vi "Calibrate Stereo Vision System.vi"() -> ()   [LabVIEW 2019]
doc: "This example acquires images and demonstrates the binocular stereo vision algorithms installed with NI Vision Development Module. This example requires NI-IMAQdx. Refer to the Detailed Help for more information."
uses:
  SubVIs/Stereo - Calibration Manager Function.ctl
  <vilib>/vision/Stereo.llb/IMAQ Binocular Reference Coordinate System.ctl
  SubVIs/Stereo - Global Variables.vi
  <vilib>/vision/NI_Vision_Development_Module.lvlib
panel:
  in  "Process Band":bool
  out "Unit":string
  in  "Units":string[](array[string])=["", "Angström", "Micrometer", "Millimeter", "Centimeter", "Meter", "Kilometer", "Microinch", "Inch", "Feet", "Nautical miles", "Standard miles", "Steps"]
  out "Depth":dbl caption="Depth:"
  in  "Interpolate Disparity":bool=TRUE
  in  "Overlay Horizontal Lines":bool
  in  "View":enum16{"Acquired Images", "Rectified Images"}(ring)
  out "Grid Descriptor":cluster{"X Step":sgl, "Y Step":sgl, "Unit":T1}={"X Step"=1.0, "Y Step"=1.0, "Unit"=enum."Inch"}
  out "Grid Size":cluster{"X":i32, "Y":i32}
  in  "Live Image":bool=TRUE
  out "Calibration Status":u16(ring)
  in  "Display":enum16{"Disparity Image", "Depth Image"}(ring)
  in  "Relative Coordinate System":T2
  out "Image":sgl[][](graph) caption="Grid Coverage"
  in  "Exit":bool
  in  "Tab Control":T3(tab)
  out "Grid Coverage":T5
  in  "Save Single Calibrations":bool
  out "Quality":T6 caption="Stereo Calibration Quality" {"Rectification Quality 2" format="%#.5g"; "Rectification Quality" format="%#.5g"; "Calibration Quality" format="%#.5g"; "Max Distance" format="%#.4g"}
  in  "Save Grid Images":bool
  out "Scrollbar":u8(slide) caption="Acquire image in..." max=50 scale=0.0..100.0
  in  "Save Stereo Calibration":bool
  in  "Scaling Factor":sgl=1.0 min=0 max=1 step=0.1
  in  "Load":bool
  in  "Calibrate":bool
  out "Instruction Images":u16(ring) caption="Grid Orientation"
  out "Instructions":string
  in  "Time Lapse":u16=4 caption="Image Acquisition Time Lapse" min=1 max=60 step=1
  out "Grid Valid":bool=TRUE
  out "Calibration Grids":cluster{"Left Image":T4, "Right Image":T4}[](array[cluster]) caption="Left Calibration Grids"
  in  "Show":enum16{"Grid Coverage", "Calibration Grids"}(ring)
  in  "Max Depth (SGBM)":sgl=45.0 caption="Maximum Depth"
  in  "Correspondence Options SGBM":T7={"Method"=0, "Window Size"=15.0, "Minimum Disparity"=0.0, "Number of Disparity"=144.0, "P1"=100.0, "P2"=500.0, "Full DP"=FALSE, "Max Left Right Disparity"=5.0, "Subpixel"=TRUE, "Invalid Disparity Replace Value"=-16.0} caption="Correspondence Options" {"Method" items=["SAD"]; "Number of Disparity" min=16.0 step=16.0; "Window Size" min=5.0 max=255.0 step=2.0}
  in  "Postfilter Options SGBM":T8={"Texture Threshold"=0.0, "Uniqueness Ratio"=0.0, "Speckle Window Size"=5.0, "Speckle Range"=200.0} caption="Postfilter Options" {"Speckle Range" min=0.0; "Speckle Window Size" min=0.0; "Uniqueness Ratio" min=0.0 max=100.0; "Texture Threshold" min=0.0}
  in  "Filter Cap":u32=32
  in  "Correspondence Options BM":T9={"Method"=0, "Window Size"=25.0, "Minimum Disparity"=0.0, "Number of Disparity"=144.0, "Left - Right Check"=5.0, "Subpixel"=TRUE, "Invalid Disparity Replace Value"=-16.0} caption="Correspondence Options" {"Method" items=["SAD"]; "Number of Disparity" min=16.0 step=16.0; "Window Size" min=5.0 max=255.0 step=2.0}
  in  "Postfilter Options BM":T8={"Texture Threshold"=0.0, "Uniqueness Ratio"=0.0, "Speckle Window Size"=5.0, "Speckle Range"=200.0} caption="Postfilter Options" {"Speckle Range" min=0.0; "Speckle Window Size" min=0.0; "Uniqueness Ratio" min=0.0 max=100.0 step=1.0; "Texture Threshold" min=0.0}
  in  "Prefilter Options":T10={"Filter Type"=2, "Filter Size"=9.0, "Filter Cap"=31.0} {"Filter Type" items=["None", "Normal Response", "Sobel"]; "Filter Cap" min=1.0 max=63.0 step=1.0; "Filter Size" min=5.0 max=255.0 step=2.0}
  in  "Max Depth (BM)":sgl=45.0 caption="Maximum Depth"
  out "Right Image":T4(plugin-control)
  out "Left Image":T4(plugin-control)
  # "Overview: Demonstrate how to calibrate a stereo system and compute a depth image.\nRequirements: LabVIEW Full Development System, NI-IMAQdx and Vision Development Module\nNote: This example does not run on LabVIEW Real Time"
  # "s"
  # "Right Calibration Grids"
  # "Set the Maximum Depth corresponding to your setting:"
  # "Set the Maximum Depth corresponding to your setting:"
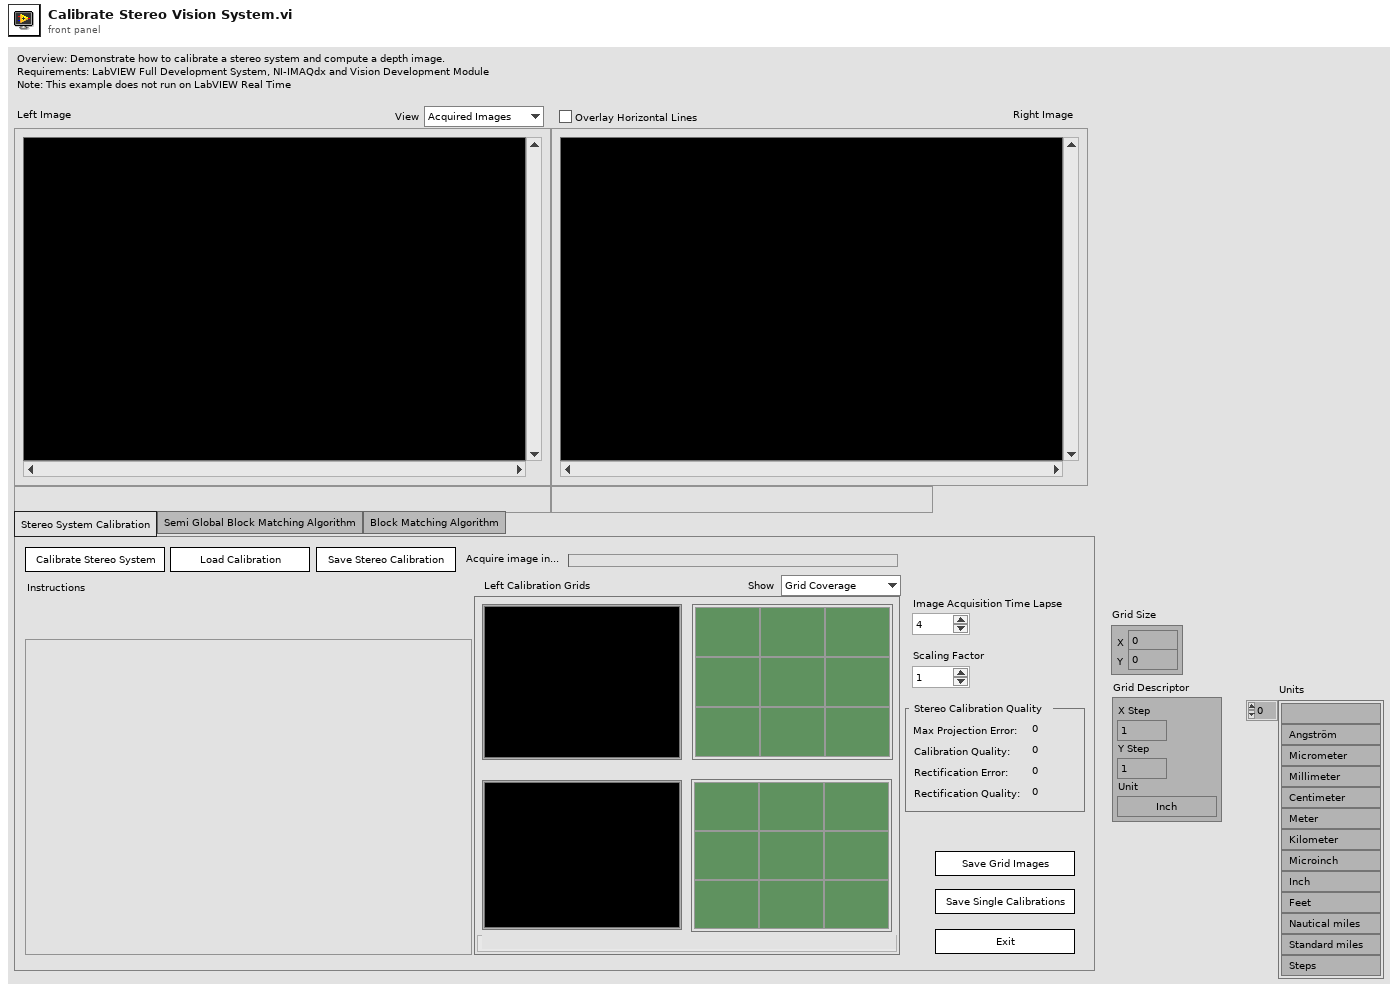
[diagram p1: front panel]
types:
  T1 = typedef "Image Unit" = enum32{"Undefined", "Angström", "Micrometer", "Millimeter", "Centimeter", "Meter", "Kilometer", "Microinch", "Inch", "Feet", "Nautical miles", "Standard miles", "Steps"}
  T2 = cluster{"Translation":cluster{"X":dbl, "Y":dbl, "Z":dbl}, "Rotation":cluster{"X":dbl, "Y":dbl, "Z":dbl}}
  T3 = enum32{"Stereo System Calibration", "Semi Global Block Matching Algorithm", "Block Matching Algorithm"}
  T4 = typedef "IMAQ Image.ctl" = refnum<image>
  T5 = cluster{"Left Image":T4, "Left Grid Coverage":bool[][], "Left Grid Coverage 3":string[][], "Right Image":T4, "Left Grid Coverage 2":bool[][], "Left Grid Coverage 4":string[][]}
  T6 = cluster{"Max Distance":dbl, "Calibration Quality":dbl, "Rectification Quality":dbl, "Rectification Quality 2":dbl}
  T7 = cluster{"Method":u16, "Window Size":dbl, "Minimum Disparity":dbl, "Number of Disparity":dbl, "P1":dbl, "P2":dbl, "Full DP":bool, "Max Left Right Disparity":dbl, "Subpixel":bool, "Invalid Disparity Replace Value":dbl}
  T8 = cluster{"Texture Threshold":dbl, "Uniqueness Ratio":dbl, "Speckle Window Size":dbl, "Speckle Range":dbl}
  T9 = cluster{"Method":u16, "Window Size":dbl, "Minimum Disparity":dbl, "Number of Disparity":dbl, "Left - Right Check":dbl, "Subpixel":bool, "Invalid Disparity Replace Value":dbl}
  T10 = cluster{"Filter Type":u16, "Filter Size":dbl, "Filter Cap":dbl}
  T11 = typedef "Stereo - Calibration Manager Function.ctl" = enum16{"Init", "Add Grid Images", "Get Images", "Dispose"}
  T12 = enum32{"Zero Order", "Bilinear", "Quadratic", "Cubic", "Bilinear Fixed"}
  T13 = typedef "IMAQ Binocular Reference Coordinate System.ctl" = enum32{" Left Camera", "Right Camera"}
  T14 = cluster{"Learn Lookup Table?":bool, "Render to original image?":bool, "Scaling Factor":sgl}
  T15 = enum8{"Enabled", "Disabled", "Disabled and Grayed Out"}
  T16 = enum32{"Page Enabled", "Page Disabled", "Page Disabled & Grayed"}
  T17 = typedef "Image Type" = u32
  T18 = typedef "IMAQ Binocular Stereo Session.ctl" = refnum<k1>
  T19 = typedef "Calibration Reference Points.ctl" = cluster{"Pixel Coordinates":cluster{"X":dbl, "Y":dbl}[], "Real World Coordinates":cluster{"X":dbl, "Y":dbl}[], "Unit":T1, "Image Size":cluster{"X":u32, "Y":u32}}
  T20 = cluster{"Image (dup)":T4, "Reference Points":T19}
  T21 = cluster{"Max. Projection Error":dbl, "Calibration Quality":dbl, "Max. Rectification Error":dbl, "Rectification Quality":dbl}
  T22 = typedef "LVPoint32TypeDef.ctl" = cluster{"Horizontal":i32, "Vertical":i32}
  T23 = cluster{"Max Depth (BM)":sgl, "Max Depth (BM)":sgl}
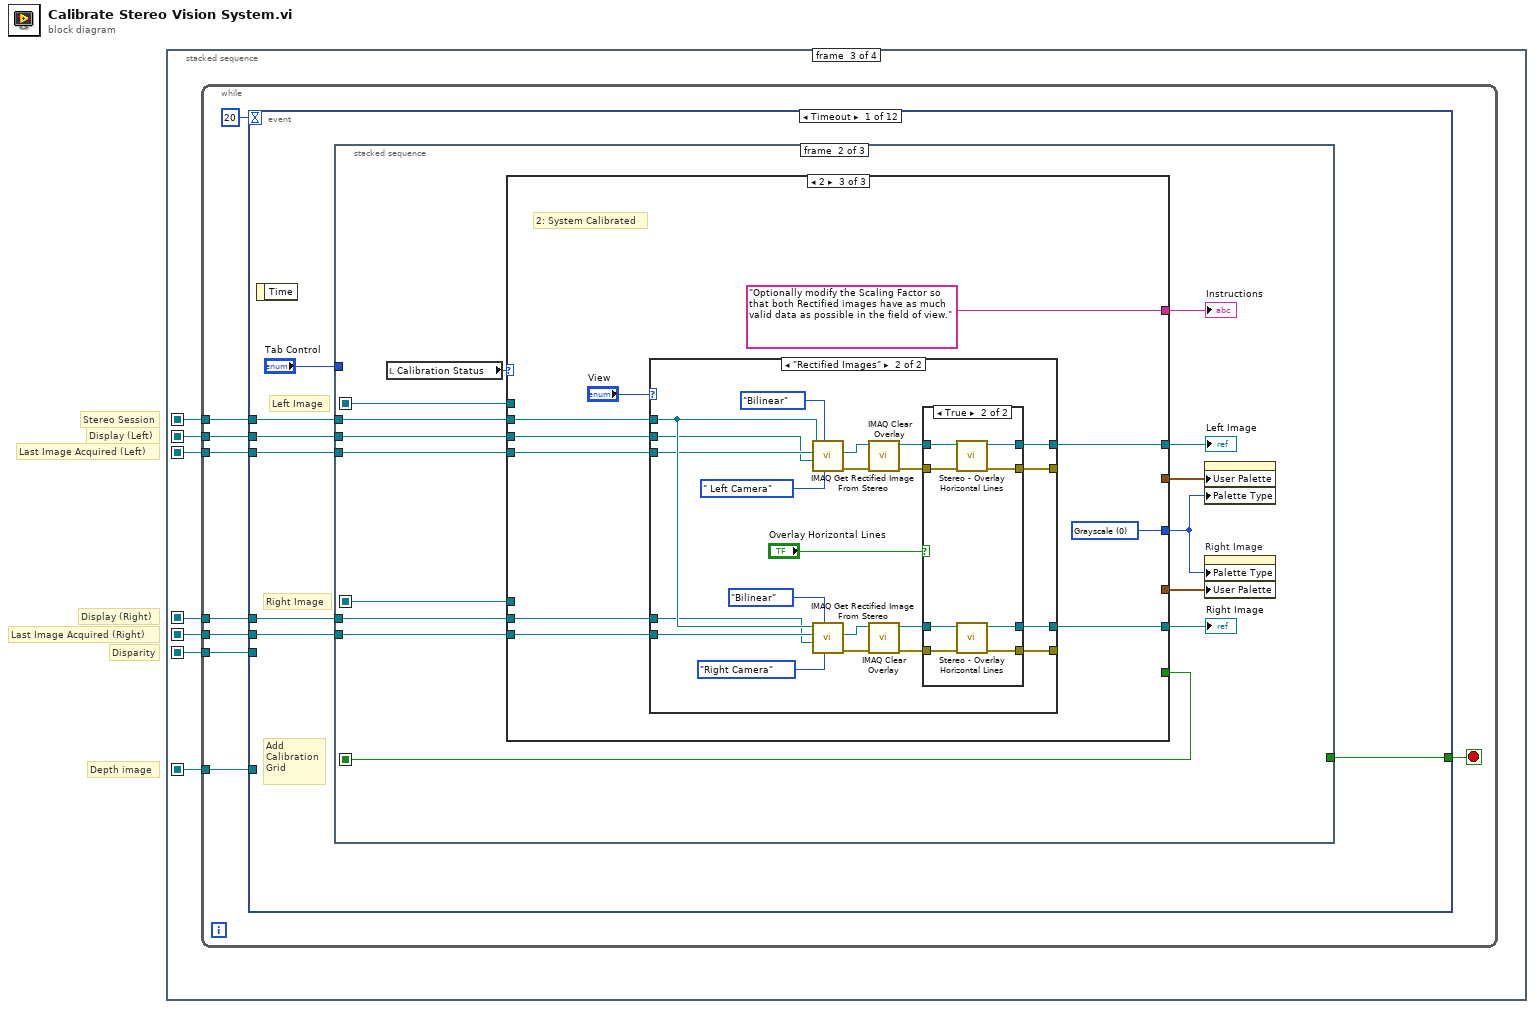
[diagram p0: block diagram]
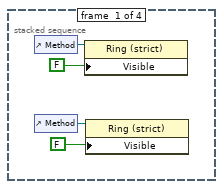
[diagram p2: hidden frame]
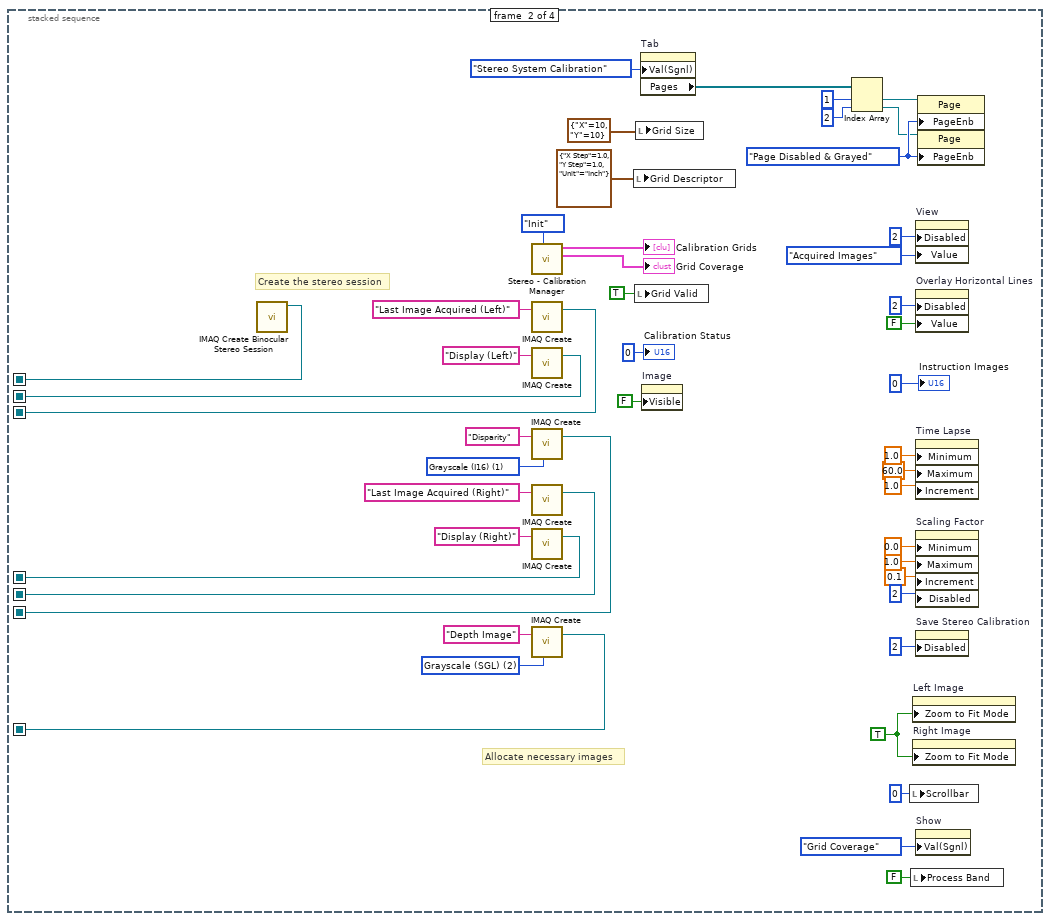
[diagram p3: hidden frame]
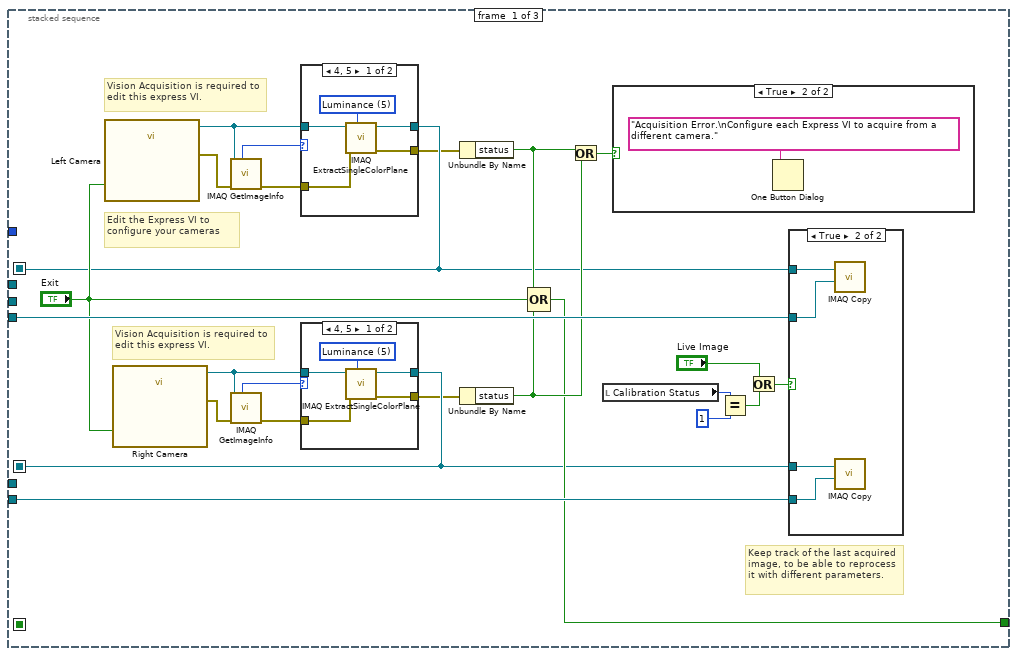
[diagram p4: hidden frame]
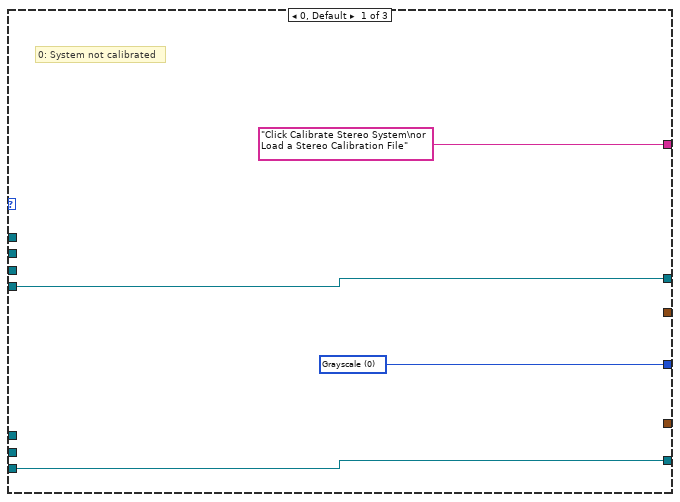
[diagram p9: hidden frame]
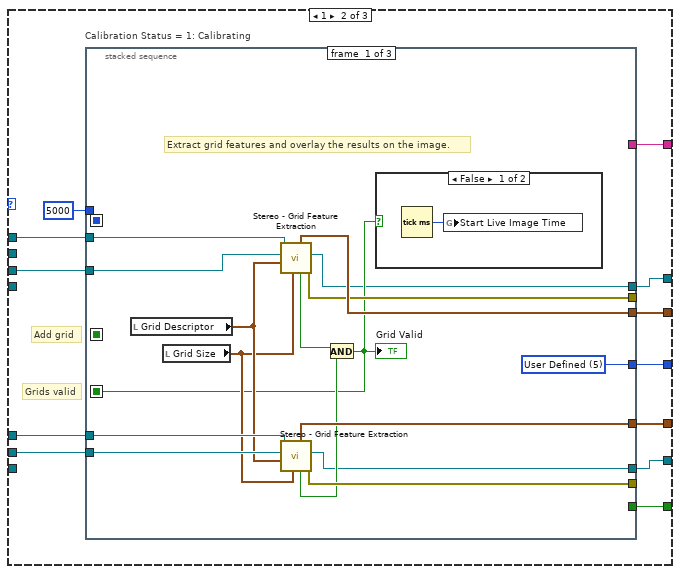
[diagram p10: hidden frame]
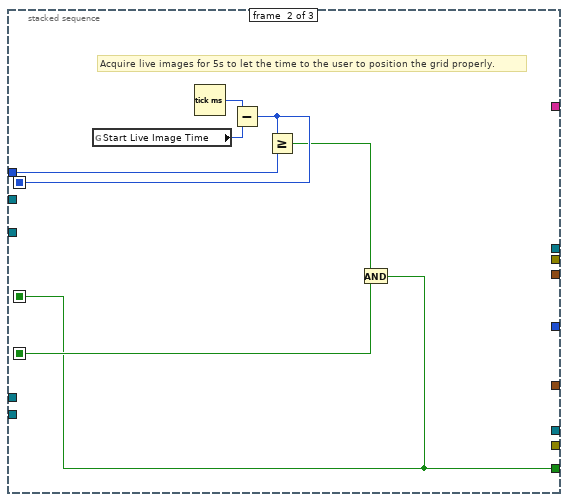
[diagram p12: hidden frame]
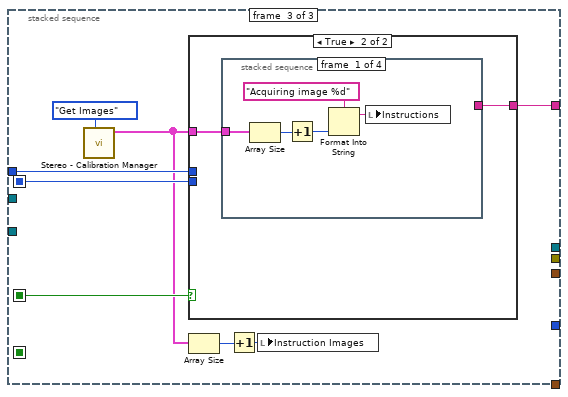
[diagram p13: hidden frame]
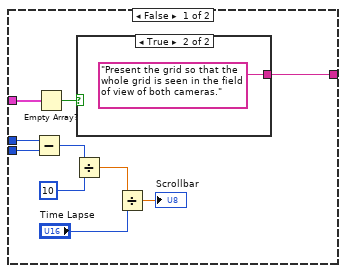
[diagram p14: hidden frame]
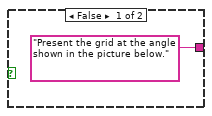
[diagram p15: hidden frame]
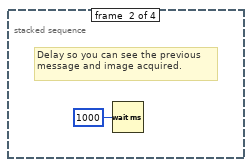
[diagram p16: hidden frame]
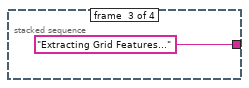
[diagram p17: hidden frame]
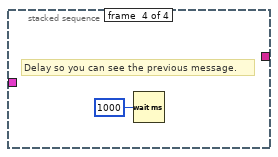
[diagram p18: hidden frame]
diagram:
  # "Depth image"
  # "Last Image Acquired (Right)"
  # "Disparity"
  # "Display (Right)"
  # "Display (Left)"
  # "Last Image Acquired (Left)"
  # "Stereo Session"
  n1 = stacked-sequence {
    seq-local: [_ w49 _ _] -> [_ _ w58 w606]
    seq-local: [_ w48 _ _] -> [_ _ w57 w604]
    seq-local: [_ w47 _ _] -> [_ _ w56 w607]
    seq-local: [_ w42 _ _] -> [_ _ w54 w603]
    seq-local: [_ w43 _ _] -> [_ _ w55 w605]
    seq-local: [_ w40 _ _] -> [_ _ w53 w602]
    seq-local: [_ w36 _ _] -> [_ _ w52 w600]
    frame #0 {
      n2 = control-ref of="Method"() -> (w4:refnum<vi>)
      n3 = control-ref of="Method"() -> (w1:refnum<vi>)
      n4 = property class="Ring (strict)"(reference=w4, "Visible"=FALSE) -> ()  [unwired: 1 in, 2 out]
      n5 = property class="Ring (strict)"(reference=w1, "Visible"=FALSE) -> ()  [unwired: 1 in, 2 out]
    }
    frame #1 {
      w12 = TRUE ("Zoom to Fit Mode")
      w30 = T16."Page Disabled & Grayed" ("Page Enabled State")
      w37 = T17 2 items=["Grayscale (U8)", "Grayscale (I16)", "Grayscale (SGL)", "Complex (CSG)", "RGB (U32)", "HSL (U32)", "RGB (U64)", "Grayscale (U16)"] ("Image Type")
      w39 = T17 1 items=["Grayscale (U8)", "Grayscale (I16)", "Grayscale (SGL)", "Complex (CSG)", "RGB (U32)", "HSL (U32)", "RGB (U64)", "Grayscale (U16)"] ("Image Type")
      # "Allocate necessary images"
      # "Create the stereo session"
      n6 = call "IMAQ Create Binocular Stereo Session"() -> ("Binocular Stereo Session Out"=w47:T18)  [unwired: 1 in, 10 out]
      n7 = call "Stereo - Calibration Manager.vi"("Function"=Stereo_-_Calibration_Manager_Function."Init") -> ("Grid Coverage"=→"Grid Coverage":T5, "Grid Images out"=→"Calibration Grids":cluster{"Left Image":T4, "Right Image":T4}[])  [unwired: 2 in, 7 out]
      n8 = call "IMAQ Create"("Image Name"="Last Image Acquired (Left)") -> ("New Image"=w43:T4)  [unwired: 3 in, 2 out]
      n9 = call "IMAQ Create"("Image Name"="Display (Left)") -> ("New Image"=w49:T4)  [unwired: 3 in, 2 out]
      n10 = call "IMAQ Create"("Image Name"="Disparity", "Image Type"=w39) -> ("New Image"=w40:T4)  [unwired: 2 in, 2 out]
      n11 = call "IMAQ Create"("Image Name"="Last Image Acquired (Right)") -> ("New Image"=w42:T4)  [unwired: 3 in, 2 out]
      n12 = call "IMAQ Create"("Image Name"="Display (Right)") -> ("New Image"=w48:T4)  [unwired: 3 in, 2 out]
      n13 = call "IMAQ Create"("Image Name"="Depth Image", "Image Type"=w37) -> ("New Image"=w36:T4)  [unwired: 2 in, 2 out]
      n14 = local write "Grid Descriptor"(cluster{"X Step":sgl, "Y Step":sgl, "Unit":T1} {"X Step"=1.0, "Y Step"=1.0, "Unit"=enum."Inch"} ("Grid Descriptor")) -> ()
      n15 = local write "Grid Valid"(TRUE ("Grid Valid")) -> ()
      n16 = local write "Grid Size"(cluster{"X":i32, "Y":i32} {"X"=10, "Y"=10} ("Grid Size")) -> ()
      n17 = property on="Tab" class="TabCtl (strict)"("Val(Sgnl)"=T3."Stereo System Calibration" ("Value (Signaling)")) -> ("Pages"=w34:refnum<vi>[])  [unwired: 2 in, 2 out]
      n18 = property on="Image" class="IntGraph (strict)"("Visible"=FALSE) -> ()  [unwired: 2 in, 2 out]
      n19 = Index Array(array=w34, index #1=1 ("index"), index #2=2 ("index")) -> (element #1=w33:refnum<vi>, element #2=w29:refnum<vi>)
      n20 = local write "Scrollbar"(u8 0 ("Scrollbar")) -> ()
      n21 = local write "Process Band"(FALSE ("Process Band")) -> ()
      n22 = property on="Left Image" class="ImageControl"("Zoom to Fit Mode"=w12) -> ()  [unwired: 2 in, 2 out]
      n23 = property on="Right Image" class="ImageControl"("Zoom to Fit Mode"=w12) -> ()  [unwired: 2 in, 2 out]
      n24 = property on="View" class="Enum (strict)"("Disabled"=u8 2, "Value"=enum16{"Acquired Images", "Rectified Images"}."Acquired Images" ("View")) -> ()  [unwired: 2 in, 2 out]
      n25 = property on="Overlay Horizontal Lines" class="Bool (strict)"("Disabled"=u8 2, "Value"=FALSE ("Overlay Horizontal Lines")) -> ()  [unwired: 2 in, 2 out]
      n26 = property on="Time Lapse" class="DigNum (strict)"("Minimum"=1.0 ("Data Entry Limits:Minimum"), "Maximum"=60.0 ("Data Entry Limits:Maximum"), "Increment"=1.0 ("Data Entry Limits:Increment")) -> ()  [unwired: 2 in, 2 out]
      n27 = property on="Scaling Factor" class="DigNum (strict)"("Minimum"=0.0 ("Data Entry Limits:Minimum"), "Maximum"=1.0 ("Data Entry Limits:Maximum"), "Increment"=0.1 ("Data Entry Limits:Increment"), "Disabled"=u8 2) -> ()  [unwired: 2 in, 2 out]
      n28 = property on="Save Stereo Calibration" class="Bool"("Disabled"=u8 2) -> ()  [unwired: 2 in, 2 out]
      n29 = property on="Show" class="Enum (strict)"("Val(Sgnl)"=enum16{"Grid Coverage", "Calibration Grids"}."Grid Coverage" ("Value (Signaling)")) -> ()  [unwired: 2 in, 2 out]
      n30 = property class="Page"(reference=w33, "PageEnb"=w30) -> ()  [unwired: 1 in, 2 out]
      n31 = property class="Page"(reference=w29, "PageEnb"=w30) -> ()  [unwired: 1 in, 2 out]
      "Calibration Status" <- u16 0 ("Status")
      "Instruction Images" <- u16 0 ("Grid Orientation")
    }
    frame #2 {
      n32 = while {
        tunnel: w58 -> [w66]
        tunnel: w57 -> [w65]
        tunnel: w56 -> [w63]
        tunnel: w55 -> [w62]
        tunnel: w54 -> [w61]
        tunnel: w53 -> [w60]
        tunnel: w52 -> [w59]
        stop <- w67 stop-if-true
        n33 = event shown="[0] Timeout" {
          selector: _ -> [_ _ _ _ _ _ _ _ _ _ _ _]
          dyn-events: _ -> [_ _ _ _ _ _ _ _ _ _ _ _]
          timeout: 20 -> [_ _ _ _ _ _ _ _ _ _ _ _]
          tunnel: [w74 _ _ _ _ _ _ _ _ _ _ _] -> w67
          tunnel: w66 -> [w73 _ _ _ _ _ _ _ _ _ _ _]
          tunnel: w65 -> [w72 _ _ _ _ _ _ _ _ _ _ _]
          tunnel: w63 -> [w69 _ _ w328 w377 w391 _ _ _ w455 _ w591]
          tunnel: w62 -> [w71 _ _ _ _ _ _ _ _ w454 _ _]
          tunnel: w61 -> [w70 _ _ _ _ _ _ _ _ w453 _ _]
          tunnel: w60 -> [_ _ _ _ _ _ _ _ _ w452 _ w590]
          tunnel: w59 -> [_ _ _ _ _ _ _ _ _ w445 _ _]
          event Timeout {
            # "Add\nCalibration\nGrid"
            # "Right Image"
            # "Left Image"
            n34 = event-data() -> ()  [unwired: 2 out]
            n35 = stacked-sequence {
              seq-local: [w82 _ _] -> [_ w129 w254]
              seq-local: [w77 _ _] -> [_ w127 w253]
              seq-local: [_ w131 _] -> [_ _ w250]
              tunnel: [w87 _ _] -> w74
              tunnel: w73 -> [_ w128 w252]
              tunnel: w72 -> [_ w126 w251]
              tunnel: w71 -> [w98 w120 _]
              tunnel: w70 -> [w97 w119 _]
              tunnel: w69 -> [_ w118 _]
              tunnel: "Tab Control" -> [_ _ w249]
              frame #0 {
                # "Vision Acquisition is required to edit this express VI."
                # "Vision Acquisition is required to edit this express VI."
                # "Edit the Express VI to configure your cameras"
                # "Keep track of the last acquired image, to be able to reprocess it with different parameters."
                n36 = call "Left Camera"("Stop (F)"="Exit") -> ("Image Out"=w83:T4, "error out"=w86:errorcluster)  [unwired: 1 in, 24 out]
                n37 = call "Right Camera"("Stop (F)"="Exit") -> ("Image Out"=w78:T4, "error out"=w85:errorcluster)  [unwired: 1 in, 24 out]
                n38 = call "IMAQ GetImageInfo"("error in (no error)"=w86, "Image"=w83) -> ("error out"=w81:errorcluster, "Image Type"=w84:T17)  [unwired: 8 out]
                n39 = call "IMAQ GetImageInfo"("error in (no error)"=w85, "Image"=w78) -> ("error out"=w79:errorcluster, "Image Type"=w75:T17)  [unwired: 8 out]
                n40 = case shown="4, 5" w84 {
                  tunnel: w83 -> [w110 w112]
                  tunnel: [w108 w112] -> w82
                  tunnel: w81 -> [w107 w111]
                  tunnel: [w106 w111] -> w80
                  frame 4, 5 {
                    w109 = 5 items=["Red", "Green", "Blue", "Hue", "Saturation", "Luminance", "Value", "Intensity"] ("Color Plane")
                    n41 = call "IMAQ ExtractSingleColorPlane"("Color Plane"=w109, "error in (no error)"=w107, "Image Src"=w110) -> ("error out"=w106:errorcluster, "Image Dst Out"=w108:T4)  [unwired: 1 in, 6 out]
                  }
                  frame Default {
                  }
                }
                n42 = case shown="4, 5" w75 {
                  tunnel: w78 -> [w103 w105]
                  tunnel: [w101 w105] -> w77
                  tunnel: w79 -> [w100 w104]
                  tunnel: [w99 w104] -> w76
                  frame 4, 5 {
                    w102 = 5 items=["Red", "Green", "Blue", "Hue", "Saturation", "Luminance", "Value", "Intensity"] ("Color Plane")
                    n43 = call "IMAQ ExtractSingleColorPlane"("Color Plane"=w102, "error in (no error)"=w100, "Image Src"=w103) -> ("error out"=w99:errorcluster, "Image Dst Out"=w101:T4)  [unwired: 1 in, 6 out]
                  }
                  frame Default {
                  }
                }
                n44 = Unbundle By Name(w80) -> ("status"=w89:bool)
                n45 = Unbundle By Name(w76) -> ("status"=w88:bool)
                n46 = Compound Arithmetic op=OR(w89, "Exit", w88) -> (w87:bool)
                n47 = Or(x=w89, y=w88) -> (x .or. y?=w91:bool)
                n48 = local read "Calibration Status"() -> (w96:u16)
                n49 = case shown="True" w91 {
                  frame False {
                  }
                  frame True {
                    n50 = One Button Dialog(message="Acquisition Error.\nConfigure each Express VI to acquire from a different camera.") -> ()  [unwired: 2 out]
                  }
                }
                n51 = Equal?(x=w96, y=u16 1) -> (x = y?=w93:bool)
                n52 = Or(x="Live Image", y=w93) -> (x .or. y?=w92:bool)
                n53 = case shown="True" w92 {
                  tunnel: w82 -> [_ w117]
                  tunnel: w98 -> [_ w116]
                  tunnel: w77 -> [_ w115]
                  tunnel: w97 -> [_ w114]
                  frame False {
                  }
                  frame True {
                    n54 = call "IMAQ Copy"("Image Dst"=w116, "Image Src"=w117) -> ()  [unwired: 1 in, 5 out]
                    n55 = call "IMAQ Copy"("Image Dst"=w114, "Image Src"=w115) -> ()  [unwired: 1 in, 5 out]
                  }
                }
              }
              frame #1 {
                n56 = local read "Calibration Status"() -> (w130:u16)
                n57 = case shown="2" w130 {
                  tunnel: ["Click Calibrate Stereo System\nor Load a Stereo Calibration File" ("Instructions") w148 "Optionally modify the Scaling Factor so that both Rectified images have as much valid data as possible in the field of view." ("Instructions")] -> w132
                  tunnel: [_ w147 _] -> w131
                  tunnel: w129 -> [_ w146 _]
                  tunnel: w128 -> [_ w145 w205]
                  tunnel: w127 -> [_ w144 _]
                  tunnel: w126 -> [_ w143 w204]
                  tunnel: [w135 w142 w209] -> w122
                  tunnel: [w134 w141 w207] -> w123
                  tunnel: [_ w140 _] -> w125
                  tunnel: [_ w139 _] -> w124
                  tunnel: [w136 w138 w212] -> w121
                  tunnel: w120 -> [w135 _ w210]
                  tunnel: w119 -> [w134 _ w208]
                  tunnel: w118 -> [_ _ w206]
                  frame 0, Default {
                    w136 = u32 0 items=["Grayscale", "Binary", "Gradient", "Rainbow", "Temperature", "User Defined"] ("Palette:Palette Type")
                    # "0: System not calibrated"
                  }
                  frame 1 {
                    # "Add grid"
                    # "Grids valid"
                    n58 = stacked-sequence "Calibration Status = 1: Calibrating" {
                      seq-local: [w151 _ _] -> [_ w167 _]
                      seq-local: [_ w166 _] -> [_ _ w180]
                      seq-local: [_ w169 _] -> [_ _ w178]
                      tunnel: [_ _ w177] -> w148
                      tunnel: [_ w166 _] -> w147
                      tunnel: w146 -> [w164 _ _]
                      tunnel: w145 -> [w163 _ _]
                      tunnel: w144 -> [w162 _ _]
                      tunnel: w143 -> [w161 _ _]
                      tunnel: [w150 _ _] -> w142
                      tunnel: [w149 _ _] -> w141
                      tunnel: [w160 _ _] -> w140
                      tunnel: [w159 _ _] -> w139
                      tunnel: [w158 _ _] -> w138
                      tunnel: [w157 _ _] -> _
                      tunnel: [w156 _ _] -> _
                      tunnel: u32 5000 ("y") -> [_ w170 w179]
                      frame #0 {
                        w158 = u32 5 items=["Grayscale", "Binary", "Gradient", "Rainbow", "Temperature", "User Defined"] ("Palette:Palette Type")
                        # "Extract grid features and overlay the results on the image."
                        n59 = local read "Grid Descriptor"() -> (w155:cluster{"X Step":sgl, "Y Step":sgl, "Unit":T1})
                        n60 = local read "Grid Size"() -> (w154:cluster{"X":i32, "Y":i32})
                        n61 = call "Stereo - Grid Feature Extraction.vi"("Grid Size"=w154, "Grid Descriptor"=w155, "Display Image in"=w163, "Image in"=w164) -> ("error out"=w157:errorcluster, "Display Image out"=w150:T4, "Valid Grid"=w153:bool, "Color Palette"=w159:cluster{"Red":u8, "Green":u8, "Blue":u8}[])  [unwired: 2 in, 2 out]
                        n62 = call "Stereo - Grid Feature Extraction.vi"("Grid Size"=w154, "Grid Descriptor"=w155, "Display Image in"=w161, "Image in"=w162) -> ("error out"=w156:errorcluster, "Display Image out"=w149:T4, "Valid Grid"=w152:bool, "Color Palette"=w160:cluster{"Red":u8, "Green":u8, "Blue":u8}[])  [unwired: 2 in, 2 out]
                        n63 = And(x=w153, y=w152) -> (x .and. y?=w151:bool)
                        "Grid Valid" <- w151
                        n64 = case shown="False" w151 {
                          frame False {
                            n65 = Tick Count (ms)() -> (millisecond timer value=w165:u32)
                            n66 = global write "Stereo - Global Variables.vi" "Start Live Image Time"(w165) -> ()
                          }
                          frame True {
                          }
                        }
                      }
                      frame #1 {
                        # "Acquire live images for 5s to let the time to the user to position the grid properly."
                        n67 = global read "Stereo - Global Variables.vi" "Start Live Image Time"() -> (w171:u32)
                        n68 = Tick Count (ms)() -> (millisecond timer value=w172:u32)
                        n69 = Subtract(x=w172, y=w171) -> (x-y=w169:u32)
                        n70 = Greater Or Equal?(x=w169, y=w170) -> (x >= y?=w168:bool)
                        n71 = And(x=w168, y=w167) -> (x .and. y?=w166:bool)
                      }
                      frame #2 {
                        n72 = call "Stereo - Calibration Manager.vi"("Function"=Stereo_-_Calibration_Manager_Function."Get Images") -> ("Grid Images out"=w173:cluster{"Left Image":T4, "Right Image":T4}[])  [unwired: 2 in, 8 out]
                        n73 = case shown="True" w180 {
                          tunnel: w178 -> [w189 _]
                          tunnel: w179 -> [w190 _]
                          tunnel: [w181 w194] -> w177
                          tunnel: w173 -> [w186 w193]
                          frame False {
                            n74 = Subtract(x=w190, y=w189) -> (x-y=w188:u32)
                            n75 = Empty Array?(array=w186) -> (empty?=w185:bool)
                            n76 = Divide(x=w188, y=u32 10) -> (x/y=w183:dbl)
                            n77 = case shown="True" w185 {
                              tunnel: ["Present the grid at the angle shown in the picture below." ("Instructions") "Present the grid so that the whole grid is seen in the field of view of both cameras." ("Instructions")] -> w181
                              frame False {
                              }
                              frame True {
                              }
                            }
                            n78 = Divide(x=w183, y="Time Lapse") -> (x/y=→"Scrollbar":dbl)
                          }
                          frame True {
                            n79 = stacked-sequence {
                              tunnel: [_ _ "Extracting Grid Features..." ("Instructions") _] -> w194
                              tunnel: w193 -> [w195 _ _ _]
                              frame #0 {
                                n80 = Array Size(array=w195) -> (size(s)=w199:i32)
                                n81 = Increment(x=w199) -> (x+1=w197:i32)
                                n82 = Format Into String(format string="Acquiring image %d" ("Instructions"), w197) -> (resulting string=w196:string)  [unwired: 2 in, 1 out]
                                n83 = local write "Instructions"(w196) -> ()
                              }
                              frame #1 {
                                # "Delay so you can see the previous message and image acquired."
                                n84 = Wait (ms)(milliseconds to wait=u32 1000) -> ()  [unwired: 1 out]
                              }
                              frame #2 {
                              }
                              frame #3 {
                                # "Delay so you can see the previous message."
                                n85 = Wait (ms)(milliseconds to wait=u32 1000) -> ()  [unwired: 1 out]
                              }
                            }
                          }
                        }
                        n86 = Array Size(array=w173) -> (size(s)=w175:i32)
                        n87 = Increment(x=w175) -> (x+1=w174:i32)
                        n88 = local write "Instruction Images"(w174) -> ()
                      }
                    }
                  }
                  frame 2 {
                    w212 = u32 0 items=["Grayscale", "Binary", "Gradient", "Rainbow", "Temperature", "User Defined"] ("Palette:Palette Type")
                    # "2: System Calibrated"
                    n89 = case shown="\"Rectified Images\"" "View" {
                      tunnel: w210 -> [w213 w233]
                      tunnel: [w213 w228] -> w209
                      tunnel: w208 -> [w214 w232]
                      tunnel: [w214 w227] -> w207
                      tunnel: w206 -> [_ w236]
                      tunnel: w205 -> [_ w231]
                      tunnel: w204 -> [_ w230]
                      tunnel: [_ w229] -> _
                      tunnel: [_ w226] -> _
                      frame "Acquired Images", Default {
                      }
                      frame "Rectified Images" {
                        n90 = call "IMAQ Get Rectified Image From Stereo"("Reference Coordinate System"=IMAQ_Binocular_Reference_Coordinate_System." Left Camera", "Interpolation Type"=T12."Bilinear", "Image Dst"=w231, "Image Src"=w233, "Binocular Stereo Session"=w236) -> ("error out"=w224:errorcluster, "Image Dst Out"=w222:T4)  [unwired: 1 in, 4 out]
                        n91 = call "IMAQ Get Rectified Image From Stereo"("Reference Coordinate System"=IMAQ_Binocular_Reference_Coordinate_System."Right Camera", "Interpolation Type"=T12."Bilinear", "Image Dst"=w230, "Image Src"=w232, "Binocular Stereo Session"=w236) -> ("error out"=w218:errorcluster, "Image Dst Out"=w220:T4)  [unwired: 1 in, 4 out]
                        n92 = call "IMAQ Clear Overlay"("error in (no error)"=w224, "Image"=w222) -> ("error out"=w223:errorcluster, "Image Out"=w221:T4)  [unwired: 1 in, 7 out]
                        n93 = call "IMAQ Clear Overlay"("error in (no error)"=w218, "Image"=w220) -> ("error out"=w217:errorcluster, "Image Out"=w219:T4)  [unwired: 1 in, 7 out]
                        n94 = case shown="True" "Overlay Horizontal Lines" {
                          tunnel: w223 -> [w239 w248]
                          tunnel: [w239 w247] -> w229
                          tunnel: w221 -> [w240 w246]
                          tunnel: [w240 w245] -> w228
                          tunnel: w219 -> [w238 w244]
                          tunnel: [w238 w243] -> w227
                          tunnel: w217 -> [w237 w242]
                          tunnel: [w237 w241] -> w226
                          frame False {
                          }
                          frame True {
                            n95 = call "Stereo - Overlay Horizontal Lines.vi"("error in (no error)"=w248, "Rectified Image in"=w246) -> ("error out"=w247:errorcluster, "Rectified Image out"=w245:T4)  [unwired: 1 in, 7 out]
                            n96 = call "Stereo - Overlay Horizontal Lines.vi"("error in (no error)"=w242, "Rectified Image in"=w244) -> ("error out"=w241:errorcluster, "Rectified Image out"=w243:T4)  [unwired: 1 in, 7 out]
                          }
                        }
                      }
                    }
                  }
                }
                "Instructions" <- w132
                "Left Image" <- w122
                "Right Image" <- w123
                n97 = property on="Left Image" class="ImageControl"("User Palette"=w124, "Palette Type"=w121) -> ()  [unwired: 2 in, 2 out]
                n98 = property on="Right Image" class="ImageControl"("Palette Type"=w121, "User Palette"=w125) -> ()  [unwired: 2 in, 2 out]
              }
              frame #2 {
                n99 = case shown="\"Stereo System Calibration\"" w249 {
                  tunnel: w254 -> [w259 _]
                  tunnel: w253 -> [w258 _]
                  tunnel: w252 -> [w257 _]
                  tunnel: w251 -> [w256 _]
                  tunnel: w250 -> [w255 _]
                  frame "Stereo System Calibration" {
                    n100 = case shown="True" w255 {
                      tunnel: w259 -> [_ w263]
                      tunnel: w258 -> [_ w262]
                      tunnel: w257 -> [_ w261]
                      tunnel: w256 -> [_ w260]
                      frame False {
                      }
                      frame True {
                        n101 = stacked-sequence {
                          tunnel: w263 -> [w280 _]
                          tunnel: w262 -> [w279 _]
                          tunnel: w261 -> [w278 _]
                          tunnel: w260 -> [w277 _]
                          frame #0 {
                            # "Extract the features from the grids."
                            n102 = local read "Grid Descriptor"() -> (w264:cluster{"X Step":sgl, "Y Step":sgl, "Unit":T1})
                            n103 = local read "Grid Size"() -> (w265:cluster{"X":i32, "Y":i32})
                            n104 = call "Stereo - Grid Feature Extraction.vi"("Grid Size"=w265, "Grid Descriptor"=w264, "Display Image in"=w278, "Image in"=w280) -> ("error out"=w267:errorcluster, "Reference Points"=w275:T19, "Image (dup)"=w276:T4, "Valid Grid"=w269:bool, "Color Palette"=w271:cluster{"Red":u8, "Green":u8, "Blue":u8}[])  [unwired: 2 in, 1 out]
                            n105 = call "Stereo - Grid Feature Extraction.vi"("Grid Size"=w265, "Grid Descriptor"=w264, "Display Image in"=w277, "Image in"=w279) -> ("error out"=w266:errorcluster, "Reference Points"=w273:T19, "Image (dup)"=w274:T4, "Valid Grid"=w268:bool, "Color Palette"=w270:cluster{"Red":u8, "Green":u8, "Blue":u8}[])  [unwired: 2 in, 1 out]
                            n106 = And(x=w269, y=w268) -> (x .and. y?=w272:bool)
                            n107 = case shown="True" w272 {
                              tunnel: w276 -> [_ w288]
                              tunnel: w275 -> [_ w287]
                              tunnel: w274 -> [_ w286]
                              tunnel: w273 -> [_ w285]
                              tunnel: w271 -> [_ w284]
                              tunnel: w270 -> [_ w283]
                              tunnel: w267 -> [_ _]
                              tunnel: w266 -> [_ _]
                              frame False {
                                n108 = flat-sequence {
                                frame #0 {
                                n109 = local write "Instructions"("Not Enough Dots Detected." ("Instructions")) -> ()
                                }
                                frame #1 {
                                # "Delay so you can see the message."
                                n110 = Wait (ms)(milliseconds to wait=u32 1000) -> ()  [unwired: 1 out]
                                }
                                }
                              }
                              frame True {
                                n111 = stacked-sequence {
                                seq-local: [_ _ w297 _] -> [_ _ _ w307]
                                tunnel: w288 -> [_ _ w305 _]
                                tunnel: w287 -> [_ _ w304 _]
                                tunnel: w286 -> [_ _ w302 _]
                                tunnel: w285 -> [_ _ w301 _]
                                tunnel: w284 -> [_ _ _ _]
                                tunnel: w283 -> [_ _ _ _]
                                frame #0 {
                                n112 = local write "Instructions"("Calibrating each camera..." ("Instructions")) -> ()
                                }
                                frame #1 {
                                # "Delay so you can see the instruction we just set in the previous frame."
                                n113 = Wait (ms)(milliseconds to wait=u32 500) -> ()  [unwired: 1 out]
                                }
                                frame #2 {
                                # "The grids are valid. Add them to the calibration manager and compute the camera models of each camera."
                                n114 = Bundle("Image (dup)"=w305, "Reference Points"=w304) -> (w303:T20)  [unwired: 1 out]
                                n115 = Bundle("Image (dup)"=w302, "Reference Points"=w301) -> (w300:T20)  [unwired: 1 out]
                                n116 = call "Stereo - Calibration Manager.vi"("Function"=Stereo_-_Calibration_Manager_Function."Add Grid Images", "Right Grid Image"=w300, "Left Grid Image"=w303) -> ("Calibration OK"=w297:bool, "Grid Coverage"=w291:T5, "Grid Images out"=w296:cluster{"Left Image":T4, "Right Image":T4}[])  [unwired: 6 out]
                                n117 = Array Size(array=w296) -> (size(s)=w295:i32)
                                n118 = local write "Grid Coverage"(w291) -> ()
                                n119 = Subtract(x=w295, y=2) -> (x-y=w293:i32)
                                n120 = Max & Min(x=w293, y=0) -> (max(x,y)=w299:i32)  [unwired: 1 out]
                                n121 = Build Array(w299) -> (w298:i32[])
                                n122 = property on="Calibration Grids" class="Arr (strict)"("Val(Sgnl)"=w296, "Index Values"=w298) -> ()  [unwired: 2 in, 2 out]
                                }
                                frame #3 {
                                n123 = case "If the single camera calibrations are OK,\nfire a Scaling Factor event to compute\nthe stereo calibration" shown="True" w307 {
                                frame False {
                                }
                                frame True {
                                n124 = property on="Scaling Factor" class="DigNum (strict)"("Val(Sgnl)"="Scaling Factor") -> ()  [unwired: 2 in, 2 out]
                                }
                                }
                                }
                                }
                              }
                            }
                          }
                          frame #1 {
                            # "Reset the Start Live Image tick count to start acquiring live images again."
                            n125 = Tick Count (ms)() -> (millisecond timer value=w309:u32)
                            n126 = global write "Stereo - Global Variables.vi" "Start Live Image Time"(w309) -> ()
                          }
                        }
                      }
                    }
                  }
                  frame Default {
                    n127 = local read "Live Image"() -> (w310:bool)
                    n128 = case shown="True" w310 {
                      frame False {
                      }
                      frame True {
                        # "If we're acquiring a live image, fire this event to process it."
                        n129 = property on="Prefilter Options" class="Clust (strict)"() -> ("Value"=w311:T10)  [unwired: 2 in, 2 out]
                        n130 = property on="Prefilter Options" class="Clust (strict)"("Val(Sgnl)"=w311) -> ()  [unwired: 2 in, 2 out]
                      }
                    }
                  }
                }
              }
            }
          }
          event "Calibrate": Value Change {
            n131 = event-data() -> ()  [unwired: 2 out]
            n132 = call "Stereo - Grid Parameters Dialog.vi"() -> ("Cancel Indicator"=w312:bool, "Grid Size out"=w313:cluster{"X":i32, "Y":i32}, "Grid Descriptor out"=w314:cluster{"X Step":sgl, "Y Step":sgl, "Unit":T1})  [unwired: 9 out]
            n133 = case shown="False" w312 {
              tunnel: w314 -> [w318 _]
              tunnel: w313 -> [w319 _]
              frame False {
                w323 = u16 1  # Calibrating...
                # "Initialize calibration manager."
                n134 = Unbundle By Name(w318) -> ("Unit"=w317:T1)
                n135 = call "Stereo - Calibration Manager.vi"("Function"=Stereo_-_Calibration_Manager_Function."Init") -> ("Grid Images out"=w320:cluster{"Left Image":T4, "Right Image":T4}[])  [unwired: 2 in, 8 out]
                n136 = Tick Count (ms)() -> (millisecond timer value=w322:u32)
                n137 = Index Array(array="Units", index=w317) -> (element=→"Unit":string)
                n138 = local write "Calibration Grids"(w320) -> ()
                n139 = global write "Stereo - Global Variables.vi" "Start Calibration Time"(w322) -> ()
                n140 = global write "Stereo - Global Variables.vi" "Start Live Image Time"(w322) -> ()
                n141 = property on="Calibration Status" class="Ring (strict)"("Value"=w323, "Blinking"=TRUE) -> ()  [unwired: 2 in, 2 out]
                "Grid Size" <- w319
                "Grid Descriptor" <- w318
              }
              frame True {
              }
            }
          }
          event "Show": Value Change {
            n142 = event-data() -> ("NewVal"=w326:enum16{"Grid Coverage", "Calibration Grids"})  [unwired: 1 out]
            n143 = Equal To 0?(x=w326) -> (x = 0?=w325:bool)
            n144 = property on="Grid Coverage" class="Clust (strict)"("Visible"=w325) -> ()  [unwired: 2 in, 2 out]
          }
          event "Scaling Factor": Value Change {
            n145 = event-data() -> ("NewVal"=w327:sgl)  [unwired: 1 out]
            n146 = stacked-sequence {
              seq-local: [_ _ w340 _] -> [_ _ _ w364]
              tunnel: w328 -> [_ _ w345 _]
              tunnel: w327 -> [_ _ w341 _]
              frame #0 {
                n147 = local write "Instructions"("Computing Stereo Calibration" ("Instructions")) -> ()
              }
              frame #1 {
                # "Delay so you can see the previous message."
                n148 = Wait (ms)(milliseconds to wait=u32 1000) -> ()  [unwired: 1 out]
              }
              frame #2 {
                # "Compute the stereo vision calibration"
                n149 = call "Stereo - Calibration Manager.vi"("Function"=Stereo_-_Calibration_Manager_Function."Get Images") -> ("Calibrated Images"=w343:T4[])  [unwired: 2 in, 8 out]
                n150 = Bundle By Name(cluster=T14 {"Learn Lookup Table?"=TRUE, "Render to original image?"=FALSE, "Scaling Factor"=0.0} ("Rectification Settings"), "Scaling Factor"=w341) -> (w333:T14)
                n151 = Index Array(array=w343) -> (element #1=w332:T4, element #2=w338:T4)  [unwired: 2 in]
                n152 = call "IMAQ GetImageSize"("Image"=w332) -> ("X Resolution"=w331:i32)  [unwired: 1 in, 4 out]
                n153 = call "Stereo - Corresponding Points Dialog.vi"("Right Image in"=w338, "Left Image in"=w332) -> ("Right Image out"=w337:T4, "Left Image out"=w339:T4)  [unwired: 8 out]
                n154 = call "IMAQ Learn Binocular Stereo Calibration"("Rectification Settings"=w333, "Right Calibration Template"=w337, "Left Calibration Template"=w339, "Binocular Stereo Session"=w345) -> ("error out"=w342:errorcluster, "Quality"=w336:T21, "Binocular Stereo Session (dup)"=w335:T18)  [unwired: 1 in, 4 out]
                "Quality" <- w336
                n155 = case shown="No Error" w342 {
                  selector: w342 -> [_ w362]
                  tunnel: [w349 w361] -> w340
                  tunnel: w336 -> [w350 _]
                  tunnel: w335 -> [w347 _]
                  tunnel: w331 -> [w346 _]
                  frame No Error {
                    n156 = Unbundle(w350) -> ("Calibration Quality"=w351:dbl)  [unwired: 3 out]
                    n157 = Greater Or Equal?(x=w351, y=0.2) -> (x >= y?=w348:bool)
                    n158 = case shown="True" w348 {
                      tunnel: [w353 w360] -> w349
                      tunnel: w347 -> [_ w359]
                      tunnel: w346 -> [_ w355]
                      frame False {
                        w353 = u16 1  # Calibrating
                      }
                      frame True {
                        w360 = u16 2  # System Calibrated
                        n159 = call "IMAQ Get Binocular Stereo Calibration Info"("Binocular Stereo Session"=w359) -> ("Q Matrix"=w358:dbl[][], "error out"=w357:errorcluster)  [unwired: 1 in, 12 out]
                        n160 = call "IMAQ Get Maximum Disparity 2"("error in (no error)"=w357, "Image Width (pixels)"=w355, "Min. Desired Depth (units)"=15.0, "Q Matrix"=w358) -> ("Max. Disparity"=w356:i32)  [unwired: 5 in, 2 out]
                        n161 = property on="Number of Disparity" class="DigNum (strict)"("Value"=w356) -> ()  [unwired: 2 in, 2 out]
                        n162 = property on="Number of Disparity" class="DigNum (strict)"("Value"=w356) -> ()  [unwired: 2 in, 2 out]
                      }
                    }
                  }
                  frame Error {
                    w361 = u16 0  # System not Calibrated
                    n163 = call <vilib>:"General Error Handler.vi"("error in (no error)"=w362) -> ()  [unwired: 2 in, 13 out]
                  }
                }
                n164 = local write "Calibration Status"(w340) -> ()
              }
              frame #3 {
                n165 = case shown="2" w364 {
                  frame 0, Default {
                  }
                  frame 2 {
                    w365 = T15."Enabled" ("Disabled")
                    w368 = T16."Page Enabled" ("Page Enabled State")
                    n166 = property on="Tab" class="TabCtl (strict)"() -> ("Pages"=w372:refnum<vi>[])  [unwired: 2 in, 2 out]
                    n167 = Index Array(array=w372, index #1=1 ("index"), index #2=2 ("index")) -> (element #1=w371:refnum<vi>, element #2=w367:refnum<vi>)
                    n168 = property on="Scaling Factor" class="DigNum (strict)"("Disabled"=w365) -> ()  [unwired: 2 in, 2 out]
                    n169 = property on="Save Stereo Calibration" class="Bool"("Disabled"=w365) -> ()  [unwired: 2 in, 2 out]
                    n170 = property on="View" class="Enum (strict)"("Disabled"=w365, "Val(Sgnl)"=enum16{"Acquired Images", "Rectified Images"}."Rectified Images" ("View")) -> ()  [unwired: 2 in, 2 out]
                    n171 = property class="Page"(reference=w371, "PageEnb"=w368) -> ()  [unwired: 1 in, 2 out]
                    n172 = property class="Page"(reference=w367, "PageEnb"=w368) -> ()  [unwired: 1 in, 2 out]
                  }
                }
                n173 = property on="Calibration Status" class="Ring (strict)"("Blinking"=FALSE) -> ()  [unwired: 2 in, 2 out]
              }
            }
          }
          event "Load": Value Change {
            n174 = event-data() -> ()  [unwired: 2 out]
            n175 = call "File Dialog2"("prompt"="Select a stereo calibration file") -> ("selected path"=w376:path, "cancelled"=w375:bool, "error out"=w373:errorcluster)  [unwired: 6 in, 6 out]
            n176 = case shown="False" w375 {
              tunnel: w377 -> [w380 _]
              tunnel: w376 -> [w378 _]
              tunnel: w373 -> [_ _]
              frame False {
                n177 = call "IMAQ Read Binocular Stereo File"("File Path"=w378, "Binocular Stereo Session (optional)"=w380) -> ("error out"=w379:errorcluster)  [unwired: 1 in, 8 out]
                n178 = case shown="No Error" w379 {
                  selector: w379 -> [_ w390]
                  frame No Error {
                    w384 = T16."Page Enabled" ("Page Enabled State")
                    w389 = u16 2  # System Calibrated
                    n179 = property on="Tab" class="TabCtl (strict)"() -> ("Pages"=w388:refnum<vi>[])  [unwired: 2 in, 2 out]
                    n180 = property on="View" class="Enum (strict)"() -> ("Value"=w382:enum16{"Acquired Images", "Rectified Images"})  [unwired: 2 in, 2 out]
                    n181 = Index Array(array=w388, index #1=1 ("index"), index #2=2 ("index")) -> (element #1=w387:refnum<vi>, element #2=w383:refnum<vi>)  [unwired: 1 in, 1 out]
                    n182 = local write "Calibration Status"(w389) -> ()
                    n183 = property on="View" class="Enum (strict)"("Disabled"=T15."Enabled", "Val(Sgnl)"=w382) -> ()  [unwired: 2 in, 2 out]
                    n184 = property class="Page"(reference=w387, "PageEnb"=w384) -> ()  [unwired: 1 in, 2 out]
                    n185 = property class="Page"(reference=w383, "PageEnb"=w384) -> ()  [unwired: 1 in, 2 out]
                  }
                  frame Error {
                    n186 = call <vilib>:"General Error Handler.vi"("error in (no error)"=w390) -> ()  [unwired: 2 in, 13 out]
                  }
                }
              }
              frame True {
              }
            }
          }
          event "Save Stereo Calibration": Value Change {
            n187 = event-data() -> ()  [unwired: 2 out]
            n188 = call "File Dialog"("prompt"="Save Stereo Calibration File As...") -> ("selected path"=w393:path, "cancelled"=w392:bool)  [unwired: 6 in, 7 out]
            n189 = case shown="False" w392 {
              tunnel: w391 -> [w396 _]
              tunnel: w393 -> [w395 _]
              frame False {
                n190 = call "IMAQ Write Binocular Stereo File"("File Path"=w395, "Binocular Stereo Session"=w396) -> ()  [unwired: 3 in, 7 out]
              }
              frame True {
              }
            }
          }
          event "Save Grid Images": Value Change {
            n191 = event-data() -> ()  [unwired: 2 out]
            n192 = call "File Dialog3"("prompt"="Save Grid Images in...") -> ("selected path"=w398:path, "cancelled"=w397:bool)  [unwired: 6 in, 7 out]
            n193 = case shown="False" w397 {
              tunnel: w398 -> [w400 _]
              frame False {
                n194 = call "Stereo - Calibration Manager.vi"("Function"=Stereo_-_Calibration_Manager_Function."Get Images") -> ("Grid Images out"=w401:cluster{"Left Image":T4, "Right Image":T4}[])  [unwired: 2 in, 8 out]
                n195 = for {
                  tunnel: w401 -> [w413] mode=indexing
                  tunnel: w400 -> [w408]
                  i -> [w404]
                  n196 = Format Into String(format string="Left Grid %d.png", w404) -> (resulting string=w409:string)  [unwired: 2 in, 1 out]
                  n197 = Format Into String(format string="Right Grid %d.png", w404) -> (resulting string=w406:string)  [unwired: 2 in, 1 out]
                  n198 = Build Path(base path=w408, name or relative path=w409) -> (appended path=w405:path)
                  n199 = Build Path(base path=w408, name or relative path=w406) -> (appended path=w403:path)
                  n200 = Unbundle By Name(w413) -> ("Left Image"=w412:T4, "Right Image"=w411:T4)
                  n201 = call-poly "IMAQ Write File 2"("File Path"=w405, "Image"=w412) -> ()  [unwired: 4 in, 6 out]
                  n202 = call-poly "IMAQ Write File 2"("File Path"=w403, "Image"=w411) -> ()  [unwired: 4 in, 6 out]
                }
              }
              frame True {
              }
            }
          }
          event "Save Single Calibrations": Value Change {
            n203 = event-data() -> ()  [unwired: 2 out]
            n204 = call "File Dialog4"("prompt"="Save Single Calibration Templates in...") -> ("selected path"=w415:path, "cancelled"=w414:bool)  [unwired: 6 in, 7 out]
            n205 = case shown="False" w414 {
              tunnel: w415 -> [w419 _]
              frame False {
                n206 = call "Stereo - Calibration Manager.vi"("Function"=Stereo_-_Calibration_Manager_Function."Get Images") -> ("Calibrated Images"=w418:T4[])  [unwired: 2 in, 8 out]
                n207 = for {
                  tunnel: w419 -> [w424]
                  tunnel: w418 -> [w423] mode=indexing
                  tunnel: string[] ["Left Single Calibration Template.png", "Right Single Calibration Template.png"] -> [w421] mode=indexing
                  n208 = Build Path(base path=w424, name or relative path=w421) -> (appended path=w422:path)
                  n209 = call-poly "IMAQ Write File 2"("File Path"=w422, "Image"=w423) -> ()  [unwired: 4 in, 6 out]
                }
              }
              frame True {
              }
            }
          }
          event "View": Value Change {
            n210 = event-data() -> ("NewVal"=w426:enum16{"Acquired Images", "Rectified Images"})  [unwired: 1 out]
            n211 = Equal?(x=w426, y=enum16{"Acquired Images", "Rectified Images"}."Rectified Images" ("View")) -> (x = y?=w430:bool)
            n212 = Select(t=u8 0 ("Disabled"), s=w430, f=u8 2) -> (s? t:f=w429:u8)
            n213 = property on="Overlay Horizontal Lines" class="Bool (strict)"("Disabled"=w429) -> ()  [unwired: 2 in, 2 out]
          }
          event "Filter Cap", "Postfilter Options SGBM", "Correspondence Options SGBM", "Prefilter Options", "Postfilter Options BM", "Correspondence Options BM", "Interpolate Disparity", "Process Band": Value Change {
            n214 = event-data() -> ()  [unwired: 2 out]
            n215 = local read "Tab Control"() -> (w443:T3)
            n216 = case shown="\"Semi Global Block Matching Algorithm\", \"Block Matching Algorithm\"" w443 {
              selector: w443 -> [_ w480]
              tunnel: w455 -> [_ w461]
              tunnel: w454 -> [_ w489]
              tunnel: w453 -> [_ w488]
              tunnel: w452 -> [_ w487]
              tunnel: "Postfilter Options BM" -> [_ w486]
              tunnel: "Prefilter Options" -> [_ w485]
              tunnel: "Correspondence Options BM" -> [_ w484]
              tunnel: "Postfilter Options SGBM" -> [_ w483]
              tunnel: "Filter Cap" -> [_ w482]
              tunnel: "Correspondence Options SGBM" -> [_ w481]
              tunnel: [w456 w474] -> w433
              tunnel: w445 -> [_ w465]
              tunnel: [FALSE ("Visible") TRUE ("Visible")] -> w444
              tunnel: [FALSE ("Visible") TRUE ("Visible")] -> w431
              tunnel: ["Grid Coverage" ("Caption.Text") w464] -> w442
              tunnel: [w457 u8 0 ("Disabled")] -> w441
              tunnel: "Interpolate Disparity" -> [_ w462]
              tunnel: "Process Band" -> [_ w473]
              frame "Stereo System Calibration", Default {
                n217 = property on="View" class="Enum (strict)"() -> ("Disabled"=w457:u8)  [unwired: 2 in, 2 out]
                n218 = property on="Image" class="IntGraph (strict)"() -> ("Value"=w456:sgl[][])  [unwired: 2 in, 2 out]
              }
              frame "Semi Global Block Matching Algorithm", "Block Matching Algorithm" {
                n219 = case shown="\"Block Matching Algorithm\", Default" w480 {
                  tunnel: w461 -> [w530 w543]
                  tunnel: w489 -> [w529 w541]
                  tunnel: w488 -> [w528 w540]
                  tunnel: w487 -> [w527 w542]
                  tunnel: [w526 w539] -> w472
                  tunnel: w486 -> [w525 _]
                  tunnel: w485 -> [w524 _]
                  tunnel: w484 -> [w522 _]
                  tunnel: w483 -> [_ w538]
                  tunnel: w482 -> [_ w537]
                  tunnel: w481 -> [_ w535]
                  tunnel: [w523 w536] -> w470
                  tunnel: [w521 w534] -> w466
                  tunnel: [w520 w533] -> w471
                  tunnel: [w519 w532] -> w475
                  tunnel: w473 -> [w518 w531]
                  frame "Block Matching Algorithm", Default {
                    n220 = call "IMAQ Stereo Correspondence (Block Matching)"("Binocular Stereo Session"=w530, "Prefilter Options"=w524, "Postfilter Options"=w525, "Process Band?"=w518, "Left Image In"=w529, "Right Image In"=w528, "Disparity Image In"=w527, "Correspondence Options"=w522) -> ("Disparity Image Out"=w526:T4, "error out"=w523:errorcluster)  [unwired: 2 in, 4 out]
                    n221 = Unbundle(w522) -> ("Minimum Disparity"=w520:dbl, "Number of Disparity"=w519:dbl, "Invalid Disparity Replace Value"=w521:dbl)  [unwired: 4 out]
                  }
                  frame "Semi Global Block Matching Algorithm" {
                    n222 = call "IMAQ Stereo Correspondence (SG Block Matching)"("Binocular Stereo Session"=w543, "Filter Cap"=w537, "Postfilter Options"=w538, "Process Band?"=w531, "Left Image In"=w541, "Right Image In"=w540, "Disparity Image In"=w542, "Correspondence Options"=w535) -> ("Disparity Image Out"=w539:T4, "error out"=w536:errorcluster)  [unwired: 2 in, 4 out]
                    n223 = Unbundle(w535) -> ("Minimum Disparity"=w533:dbl, "Number of Disparity"=w532:dbl, "Invalid Disparity Replace Value"=w534:dbl)  [unwired: 7 out]
                  }
                }
                n224 = case shown="True" w462 {
                  tunnel: w472 -> [w508 w517]
                  tunnel: [w508 w516] -> w469
                  tunnel: w466 -> [_ w515]
                  tunnel: w471 -> [_ w514]
                  tunnel: w475 -> [_ w513]
                  tunnel: w470 -> [w507 w510]
                  tunnel: [w507 w509] -> w467
                  frame False {
                  }
                  frame True {
                    n225 = call "IMAQ Interpolate Disparity Image 2"("Image Src"=w517, "Minimum Disparity"=w514, "Number of Disparities"=w513, "Invalid Disparity Value"=w515, "error in (no error)"=w510, "Order"=12, "Sampling Frequency"=25) -> ("Image Dst Out"=w516:T4, "error out"=w509:errorcluster)  [unwired: 7 in]
                  }
                }
                n226 = case shown="\"Disparity Image\", Default" "Display" {
                  tunnel: [w495 w500] -> w476
                  tunnel: w469 -> [w497 w506]
                  tunnel: w461 -> [_ w505]
                  tunnel: w467 -> [w496 w504]
                  tunnel: w466 -> [_ w503]
                  tunnel: w465 -> [_ w502]
                  tunnel: ["Disparity Image" ("Caption.Text") "Depth Image" ("Caption.Text")] -> w464
                  frame "Disparity Image", Default {
                    n227 = call "IMAQ ImageToArray"("error in (no error)"=w496, "Image"=w497) -> ("Image Pixels (I16)"=w495:i16[][])  [unwired: 1 in, 5 out]
                  }
                  frame "Depth Image" {
                    n228 = call "IMAQ Get Depth Image From Stereo"("Invalid Disparity Value"=w503, "error in (no error)"=w504, "Depth Image In"=w502, "Disparity Image"=w506, "Binocular Stereo Session"=w505) -> ("error out"=w499:errorcluster, "Depth Image Out"=w501:T4)  [unwired: 2 in, 3 out]
                    n229 = call "IMAQ ImageToArray"("error in (no error)"=w499, "Image"=w501) -> ("Image Pixels (Float)"=w500:sgl[][])  [unwired: 1 in, 5 out]
                  }
                }
                n230 = local read "Process Band"() -> (w463:bool)
                n231 = case shown="False" w463 {
                  tunnel: w476 -> [w492 w493]
                  tunnel: w475 -> [w491 _]
                  tunnel: [w490 w493] -> w474
                  frame False {
                    n232 = Array Subset(array=w492, index (col)=w491) -> (w490:sgl[][])  [unwired: 3 in]
                  }
                  frame True {
                  }
                }
              }
            }
            "Image" <- w433
            n233 = property on="View" class="Enum (strict)"("Disabled"=w441) -> ("Value"=w440:enum16{"Acquired Images", "Rectified Images"})  [unwired: 2 in, 2 out]
            n234 = property on="Image" class="IntGraph (strict)"("Visible"=w444, "Caption.Text"=w442) -> ()  [unwired: 2 in, 2 out]
            n235 = property on="Live Image" class="Bool (strict)"("Visible"=w431) -> ()  [unwired: 2 in, 2 out]
            n236 = property on="Display" class="Enum (strict)"("Visible"=w431) -> ()  [unwired: 2 in, 2 out]
            n237 = property on="Relative Coordinate System" class="Clust (strict)"("Visible"=w431) -> ()  [unwired: 2 in, 2 out]
            n238 = property on="Interpolate Disparity" class="Bool (strict)"("Visible"=w431) -> ()  [unwired: 2 in, 2 out]
            n239 = property on="Process Band" class="Bool (strict)"("Visible"=w431) -> ()  [unwired: 2 in, 2 out]
            n240 = property on="Depth" class="DigNum (strict)"("Visible"=w431) -> ()  [unwired: 2 in, 2 out]
            n241 = property on="Unit" class="Str"("Visible"=w431) -> ()  [unwired: 2 in, 2 out]
            n242 = Equal?(x=enum16{"Acquired Images", "Rectified Images"}."Rectified Images" ("View"), y=w440) -> (x = y?=w438:bool)
            n243 = Select(t=u8 0 ("Disabled"), s=w438, f=u8 2) -> (s? t:f=w437:u8)
            n244 = property on="Overlay Horizontal Lines" class="Bool (strict)"("Disabled"=w437) -> ()  [unwired: 2 in, 2 out]
          }
          event "Tab Control", "Correspondence Options SGBM.Minimum Disparity", "Correspondence Options SGBM.Number of Disparity", "Correspondence Options BM.Minimum Disparity", "Correspondence Options BM.Number of Disparity", "Display", "Max Depth (SGBM)", "Max Depth (BM)": Value Change {
            n245 = event-data() -> ()  [unwired: 2 out]
            n246 = local read "Tab Control"() -> (w547:T3)
            n247 = local read "Display"() -> (w545:enum16{"Disparity Image", "Depth Image"})
            n248 = local read "Interpolate Disparity"() -> (w544:bool)
            n249 = case shown="\"Disparity Image\", Default" w545 {
              tunnel: [w553 w566] -> w550
              tunnel: w547 -> [w554 w572]
              tunnel: [w552 w568] -> w549
              tunnel: u32[] [0, 7, 15, 22, 29, 36, 44, 51, 58, 66, 73, 80, 87, 95, 102, 109, 117, 124, 131, 138, 146, 153, 160, 168, 175, 182, 189, 197, 204, 211, 219, 226, 233, 240, 248, 255, 75263, 76799, 78335, 79871, 81407, 82943, 84479, 86015, 87551, 89087, 90623, 92159, 93695, 95231, 96767, 98303, 99839, 101375, 102911, 104447, 105983, 107519, 109055, 110591, 112127, 113663, 115199, 116735, 118271, 119807, 121343, 122879, 124415, 125951, 127487, 129023, 130559, 131069, 131063, 131057, 131051, 131045, 131039, 131033, 131027, 131021, 131015, 131009, 131003, 130997, 130991, 130985, 130979, 130973, 130967, 130961, 130955, 130949, 130943, 130937, 130931, 130925, 130919, 130913, 130907, 130901, 130895, 130889, 130883, 130877, 130871, 130865, 130859, 130853, 130847, 130841, 130835, 130829, 130823, 130817, 524033, 917249, 1310465, 1703681, 2096897, 2490113, 2883329, 3276545, 3669761, 4062977, 4456193, 4849409, 5242625, 5635841, 6029057, 6422273, 6815489, 7208705, 7601921, 7995137, 8388353, 8781569, 9174785, 9568001, 9961217, 10354433, 10747649, 11140865, 11534081, 11927297, 12320513, 12713729, 13106945, 13500161, 13893377, 14286593, 14679809, 15073025, 15466241, 15859457, 16252673, 16645889, 16776449, 16774913, 16773377, 16771841, 16770305, 16768769, 16767233, 16765697, 16762625, 16761089, 16759553, 16758017, 16756481, 16754945, 16753409, 16751873, 16750337, 16748801, 16747265, 16745729, 16744193, 16742657, 16741121, 16739585, 16738049, 16736513, 16734977, 16733441, 16731905, 16730369, 16728833, 16727297, 16725761, 16724225, 16722689, 16721153, 16719617, 16718081, 16716545, 16715009, 16713473, 16711937, 16711937, 16711943, 16711949, 16711955, 16711961, 16711967, 16711973, 16711979, 16711985, 16711991, 16711997, 16712003, 16712009, 16712015, 16712021, 16712027, 16712033, 16712039, 16712045, 16712051, 16712057, 16712063, 16712069, 16712075, 16712081, 16712087, 16712093, 16712099, 16712105, 16712111, 16712117, 16712123, 16712129, 16712135, 16712141, 16712147, 16712153, 16712159, 16712165, 16712171, 16712177, 16712183, 16712189, 16581119, 16187903, 15794687, 15401471, 15008255, 14615039, 14221823, 13828607, 13435391, 13042175, 12648959, 12255743, 11862527] ("appended array") -> [w551 w565]
              tunnel: [w551 w564] -> w548
              frame "Disparity Image", Default {
                w555 = 16.0 ("y")
                n250 = case shown="\"Block Matching Algorithm\"" w554 {
                  tunnel: [w559 w562] -> w557
                  tunnel: [w558 w561] -> w556
                  frame "Semi Global Block Matching Algorithm", Default {
                    n251 = local read "Correspondence Options SGBM"() -> (w560:T7)
                    n252 = Unbundle By Name(w560) -> ("Minimum Disparity"=w559:dbl, "Number of Disparity"=w558:dbl)
                  }
                  frame "Block Matching Algorithm" {
                    n253 = local read "Correspondence Options BM"() -> (w563:T9)
                    n254 = Unbundle By Name(w563) -> ("Minimum Disparity"=w562:dbl, "Number of Disparity"=w561:dbl)
                  }
                }
                n255 = Multiply(x=w555, y=w557) -> (x*y=w553:dbl)
                n256 = Multiply(x=w556, y=w555) -> (x*y=w552:dbl)
              }
              frame "Depth Image" {
                n257 = case shown="\"Semi Global Block Matching Algorithm\", Default" w572 {
                  tunnel: ["Max Depth (SGBM)" "Max Depth (BM)"] -> w568
                  frame "Semi Global Block Matching Algorithm", Default {
                  }
                  frame "Block Matching Algorithm" {
                  }
                }
                n258 = Reverse 1D Array(array=w565) -> (reversed array=w564:u32[])
                n259 = Multiply(x=w568, y=sgl 20.0) -> (x*y=w570:sgl)
                n260 = Divide(x=w570, y=sgl 100.0) -> (x/y=w567:sgl)
                n261 = Subtract(x=w568, y=w567) -> (x-y=w566:sgl)
              }
            }
            n262 = property on="Interpolate Disparity" class="Bool (strict)"("Val(Sgnl)"=w544) -> ()  [unwired: 2 in, 2 out]
            n263 = property on="Image" class="IntGraph (strict)"("ZScale.Minimum"=w550, "ZScale.Maximum"=w549) -> ()  [unwired: 2 in, 2 out]
            n264 = property on="Image" class="IntGraph (strict)"("Color Table"=w548) -> ()  [unwired: 2 in, 2 out]
          }
          event "Image": Mouse Move {
            n265 = event-data() -> ("CtlRef"=w584:refnum<vi>, "Coords"=w583:T22)  [unwired: 1 out]
            n266 = local read "Tab Control"() -> (w588:T3)
            n267 = case shown="\"Semi Global Block Matching Algorithm\", Default" w588 {
              tunnel: [w595 w599] -> w586
              tunnel: [w593 w597] -> w580
              tunnel: [w592 w596] -> w575
              frame "Semi Global Block Matching Algorithm", Default {
                n268 = local read "Correspondence Options SGBM"() -> (w594:T7)
                n269 = Unbundle By Name(w594) -> ("Invalid Disparity Replace Value"=w592:dbl, "Number of Disparity"=w593:dbl)
                n270 = local read "Max Depth (SGBM)"() -> (w595:sgl)
              }
              frame "Block Matching Algorithm" {
                n271 = local read "Correspondence Options BM"() -> (w598:T9)
                n272 = Unbundle By Name(w598) -> ("Invalid Disparity Replace Value"=w596:dbl, "Number of Disparity"=w597:dbl)
                n273 = local read "Max Depth (BM)"() -> (w599:sgl)
              }
            }
            n274 = invoke class="IntGraph (strict)" method="Map Coords To XY"(reference=w584, "Coords"=w583) -> ("XY"=w582:cluster{"X":dbl, "Y":dbl})  [unwired: 5 in, 6 out]
            n275 = Bundle By Name(cluster=cluster{"X":dbl, "Y":dbl} {"X"=0.0, "Y"=0.0} ("y"), "X"=w580) -> (w578:cluster{"X":dbl, "Y":dbl})
            n276 = Bundle("Max Depth (BM)"=sgl 0.0, "Max Depth (BM)"=w586) -> (w585:T23)  [unwired: 1 out]
            n277 = Add(x=w582, y=w578) -> (x+y=w581:cluster{"X":dbl, "Y":dbl})
            n278 = call "IMAQ Convert Pixel To 3D Coordinates"("Binocular Stereo Session"=w591, "Relative Coordinate System"="Relative Coordinate System", "Invalid Disparity Value"=w575, "Disparity Image"=w590, "Pixel Coordinates"=w581, "Depth Control"=w585) -> ("Real World 3D Coordinates"=w577:cluster{"X":dbl, "Y":dbl, "Z":dbl})  [unwired: 2 in, 7 out]
            n279 = Unbundle By Name(w577) -> ("Z"=→"Depth":dbl)
          }
        }
      }
    }
    frame #3 {
      # "Dispose of the session and images"
      n280 = Build Array(w606, w605, w604, w603, w602, w600) -> (w601:T4[])
      n281 = for {
        tunnel: w601 -> [w608] mode=indexing
        n282 = call "IMAQ Dispose"("Image"=w608) -> ()  [unwired: 2 in, 4 out]
      }
      n283 = call "IMAQ Dispose Binocular Stereo Session"("Binocular Stereo Session"=w607) -> ()  [unwired: 1 in, 10 out]
    }
  }
